vi "(C) Save to Excel (SubVI).vi"(0 "File Path Input":path, 1 "Save (Enable/Signal)":bool, 2 "Save Interval (s)":dbl=1.0, 3 "Title Block":string[][](array[string]), 4 "Column Header Array":string[](array[string]), 5 "Data Array (Row)":string[](array[string]), 7 "File Configuration":T1={"Row Limit"=65500, "Default File Name"="Data", "New File Daily?"=TRUE, "Manual Save Interval?"=FALSE}, 9 "Change Save Location?":bool, 11 "Reset Elapsed Time":bool caption="Reset Elapsed Time?") -> (14 "File Path Output":path, 15 "Save Indicator":bool, 16 "# of Rows Saved":i32, 17 "Elapsed Time":string="00:00:00", 19 "Error Output":errorcluster)   [LabVIEW 2010]
panel:
  # "SAVE TO EXCEL SUBVI\nSave 1D Array (Row) to File"
  # "Created by Blake Otting 3/7/2007\nLast Updated 4/15/2010"
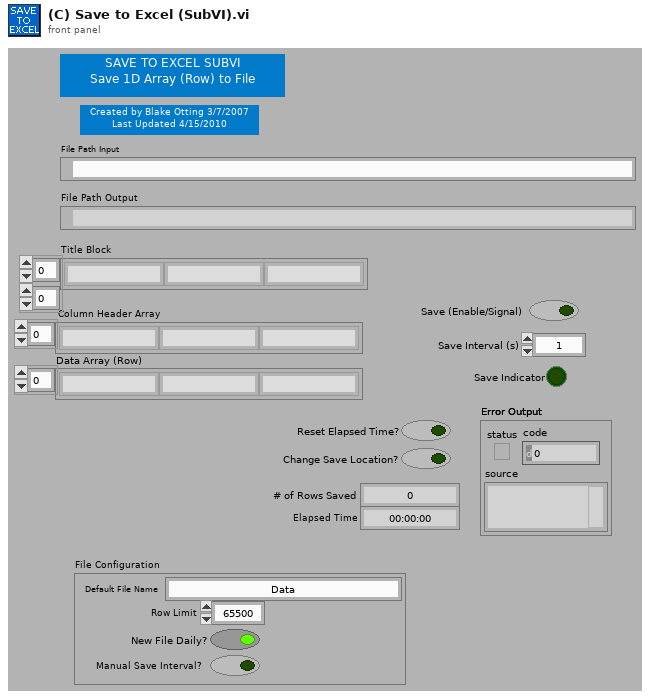
[diagram p1: front panel]
types:
  T1 = cluster{"Row Limit":i32, "Default File Name":string, "New File Daily?":bool, "Manual Save Interval?":bool}
  T2 = typedef "LVDateTimeRec.ctl" = cluster{"fractional second":dbl, "second":i32, "minute":i32, "hour":i32, "day of month":i32, "month":i32, "year":i32, "day of week":i32, "day of year":i32, "DST":i32}
  T3 = enum16{"open", "replace", "create", "open or create", "replace or create", "replace or create with confirmation"}
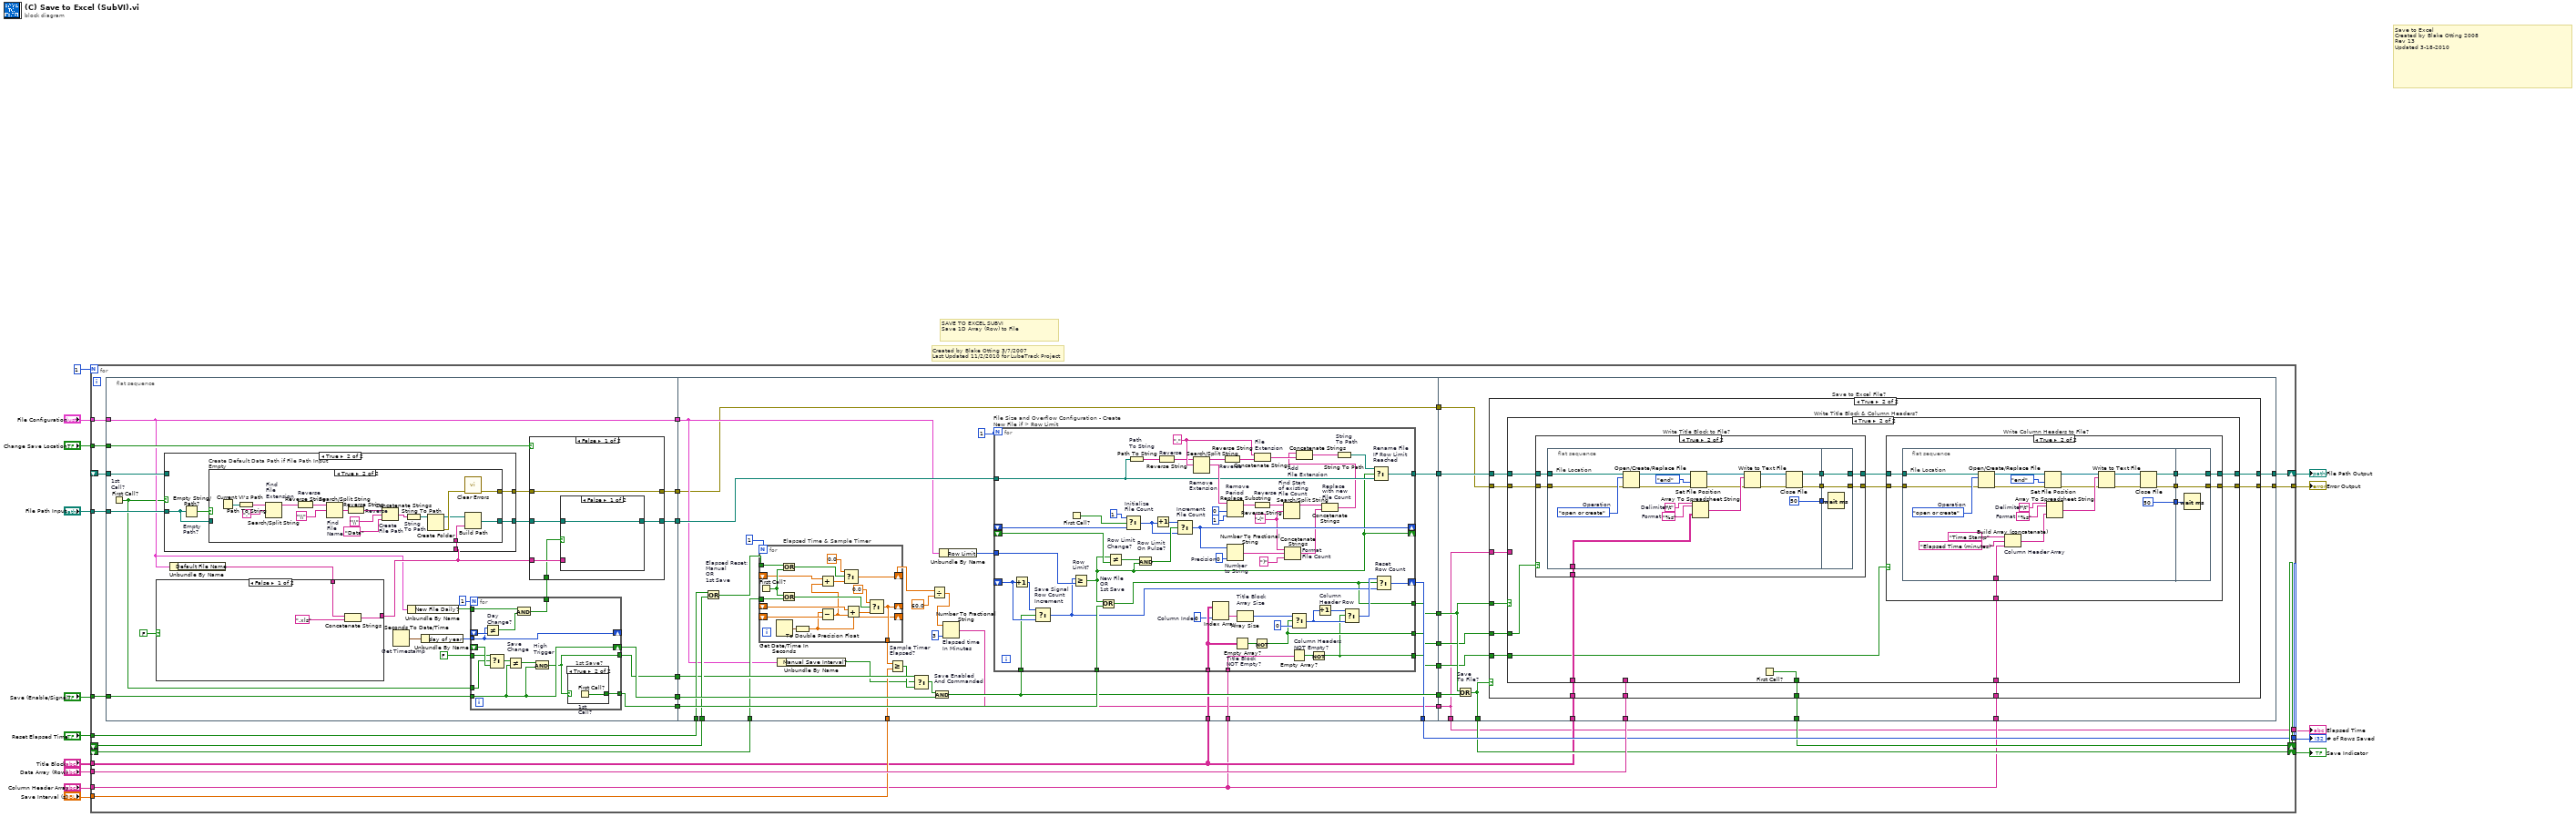
[diagram p0: block diagram]
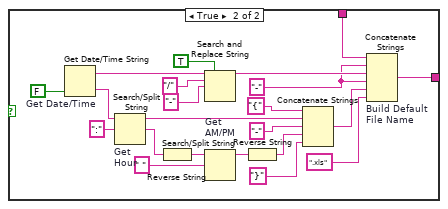
[diagram p2: hidden frame]
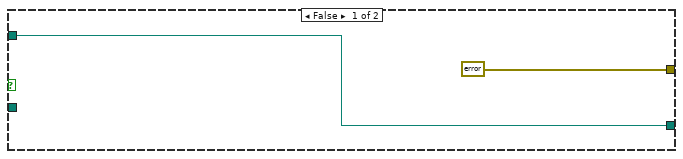
[diagram p4: hidden frame]
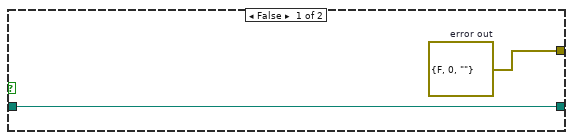
[diagram p5: hidden frame]
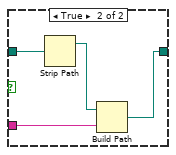
[diagram p6: hidden frame]
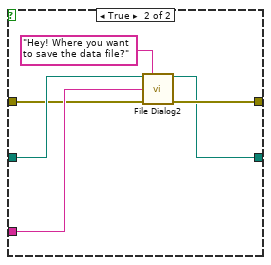
[diagram p7: hidden frame]
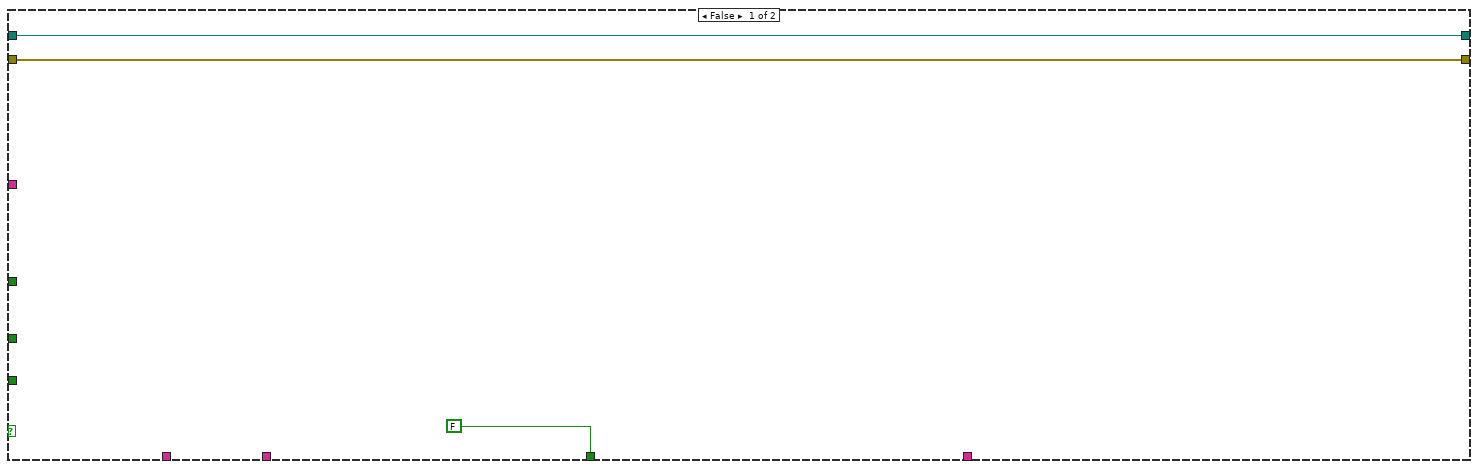
[diagram p8: hidden frame]
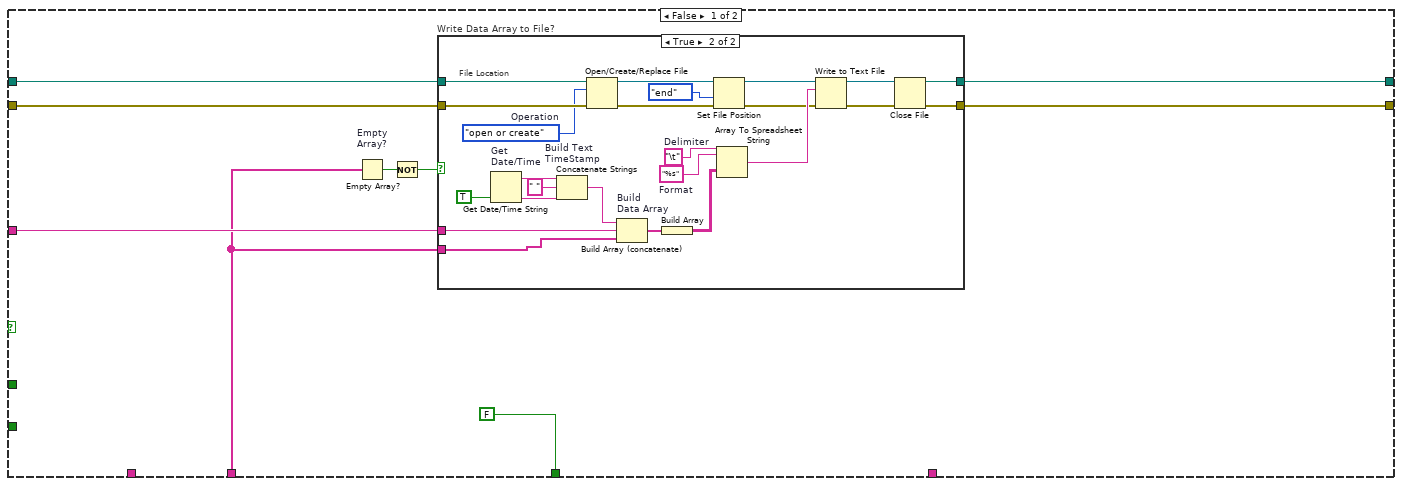
[diagram p9: hidden frame]
diagram:
  # "Created by Blake Otting 3/7/2007\nLast Updated 11/2/2010 for LubeTrack Project"
  # "SAVE TO EXCEL SUBVI\nSave 1D Array (Row) to File"
  # "Save to Excel\nCreated by Blake Otting 2008\nRev 13\nUpdated 3-18-2010"
  n1 = for {
    N: 1 -> [_]
    tunnel: "File Path Input" -> [w39]
    tunnel: "Change Save Location?" -> [w46]
    tunnel: "Save (Enable/Signal)" -> [w33]
    tunnel: "Data Array (Row)" -> [w40]
    tunnel: "Column Header Array" -> [w23]
    tunnel: "File Configuration" -> [w29]
    tunnel: "Reset Elapsed Time" -> [w30]
    shift-right: [w35] -> w14
    shift-left: _ -> [w43]
    tunnel: "Save Interval (s)" -> [w34]
    shift-right: [w36] -> _
    shift-left: _ -> [w31]
    tunnel: "Title Block" -> [w25]
    shift-right: [w41] -> w12
    shift-left: _ -> [w38]
    tunnel: [w19] -> w13
    tunnel: [w37] -> w15
    tunnel: [w26] -> w11
    n2 = flat-sequence {
      tunnel: w38 -> [w58]
      tunnel: w39 -> [w57]
      tunnel: w46 -> [w50]
      tunnel: w29 -> [w49]
      tunnel: [w52] -> w45
      tunnel: [w54] -> w44
      tunnel: w33 -> [w56]
      tunnel: [w55] -> w32
      tunnel: [w51] -> w28
      tunnel: [w49] -> w18
      tunnel: [w53] -> w17
      tunnel: [w180] -> w42
      tunnel: w43 -> [w163]
      tunnel: w44 -> [w154]
      tunnel: w45 -> [w181]
      tunnel: [w172] -> w37
      tunnel: w34 -> [w161]
      tunnel: w32 -> [w178]
      tunnel: w31 -> [w175]
      tunnel: w30 -> [w174]
      tunnel: w28 -> [w173]
      tunnel: [w154] -> w27
      tunnel: w25 -> [w171]
      tunnel: [w169] -> w24
      tunnel: w23 -> [w168]
      tunnel: [w167] -> w22
      tunnel: [w166] -> w21
      tunnel: [w159] -> w20
      tunnel: w18 -> [w158]
      tunnel: w17 -> [w170]
      tunnel: [w151] -> w16
      tunnel: w42 -> [w265]
      tunnel: [w263] -> w41
      tunnel: w25 -> [w262]
      tunnel: w40 -> [w261]
      tunnel: w23 -> [w260]
      tunnel: [w259] -> w35
      tunnel: [w258] -> w36
      tunnel: w27 -> [w257]
      tunnel: [w256] -> w26
      tunnel: w24 -> [w264]
      tunnel: w22 -> [w255]
      tunnel: w21 -> [w254]
      tunnel: w20 -> [w253]
      tunnel: [w252] -> w19
      tunnel: w16 -> [w252]
      frame #0 {
        n3 = First Call? "1st\nCall?"() -> (First Call?: T/F=w48:bool)
        n4 = Unbundle By Name(w49) -> ("Default File Name"=w60:string)
        n5 = case shown="False" FALSE {
          tunnel: [w69 w93] -> w68
          tunnel: w60 -> [w70 w92]
          frame False {
            n6 = Concatenate Strings(w70, ".xls" ("string")) -> (w69:string)
          }
          frame True {
            w81 = "-" ("string")
            n7 = Get Date/Time String "Get Date/Time"(want seconds? (F)=FALSE) -> (date string=w76:string, time string=w75:string)  [unwired: 2 out]
            n8 = Search/Split String "Get\nHour"(string=w75, search string/char (-)=":" ("search string")) -> (substring before match=w86:string, match + rest of string=w83:string)  [unwired: 2 out]
            n9 = Reverse String(1:w83) -> (0:w84:string)
            n10 = Search and Replace String(replace all?=TRUE ("replace all? (F)"), input string=w76, search string="/", replace string="-" ("replace string (\"\")")) -> (result string=w91:string)  [unwired: 1 in, 6 out]
            n11 = Search/Split String "Get\nAM/PM"(string=w84, search string/char (-)=" ") -> (substring before match=w85:string)  [unwired: 3 out]
            n12 = Reverse String(1:w85) -> (0:w87:string)
            n13 = Concatenate Strings ("Build\nHour String")("{" ("string"), w86, "-" ("search string/char (-)"), w87, "}" ("string")) -> (w78:string)
            n14 = Concatenate Strings "Build Default\nFile Name"(w92, w81, w91, w81, w78, ".xls" ("string")) -> (w93:string)
          }
        }
        n15 = case shown="True" w48 {
          tunnel: w57 -> [_ w114]
          tunnel: [w110 w113] -> w59
          tunnel: w68 -> [_ w112]
          tunnel: [errorcluster {"status"=FALSE, "code"=0, "source"=""} w111] -> w61
          tunnel: w58 -> [w110 _]
          frame False {
          }
          frame True {
            n16 = Empty String/Path? "Empty\nPath?"(string/path=w114) -> (empty?=w115:bool)
            n17 = case "Create Default Data Path if File Path Input Empty" shown="True" w115 {
              tunnel: [w117 w120] -> w113
              tunnel: w114 -> [w117 _]
              tunnel: w112 -> [_ w119]
              tunnel: [w116 w118] -> w111
              frame False {
                w116 = errorcluster {"status"=FALSE, "code"=0, "source"=""}  # error out
              }
              frame True {
                n18 = Current VI's Path() -> (path=w126:path)
                n19 = Path To String(path=w126) -> (string=w132:string)
                n20 = Search/Split String "Find\nFile \nExtension"(string=w132, search string/char (-)=".") -> (substring before match=w131:string)  [unwired: 1 in, 2 out]
                n21 = Reverse String "Reverse"(1:w131) -> (0:w130:string)
                n22 = Search/Split String "Find\nFile \nName"(string=w130, search string/char (-)="\\") -> (match + rest of string=w128:string)  [unwired: 1 in, 2 out]
                n23 = Reverse String "Reverse"(1:w128) -> (0:w127:string)
                n24 = Concatenate Strings "Create\nFile Path"(w127, "\\", "Data") -> (w134:string)
                n25 = String To Path "String\nTo Path"(string=w134) -> (path=w124:path)
                n26 = Create Folder(path (use dialog)=w124) -> (created path=w121:path, error out=w123:errorcluster)  [unwired: 2 in, 1 out]
                n27 = call <vilib>:"Clear Errors.vi"("error in (no error)"=w123) -> ("error out"=w118:errorcluster)  [unwired: 6 in]
                n28 = Build Path(base path=w121, name or relative path=w119) -> (appended path=w120:path)
              }
            }
          }
        }
        n29 = Seconds To Date/Time "Get Timestamp"() -> (date time rec=w66:T2)  [unwired: 2 out]
        n30 = Unbundle By Name(w49) -> ("New File Daily?"=w62:bool)
        n31 = Unbundle By Name(w66) -> ("day of year"=w63:i32)
        n32 = for {
          N: 1 -> [_]
          tunnel: w56 -> [w105]
          shift-right: [w105] -> w55
          shift-left: _ -> [w99]
          tunnel: w63 -> [w103]
          shift-right: [w103] -> _
          shift-left: _ -> [w104]
          tunnel: w62 -> [w101]
          tunnel: [w100] -> w65
          tunnel: [w97] -> w52
          tunnel: [w96] -> w51
          tunnel: w48 -> [w95]
          tunnel: FALSE -> [w94]
          n33 = Not Equal? "Day\nChange?"(x=w103, y=w104) -> (x != y?=w102:bool)
          n34 = Select(t=w94, s=w95, f=w99) -> (s? t:f=w98:bool)
          n35 = Not Equal? "Save\nChange"(x=w98, y=w105) -> (x != y?=w106:bool)
          n36 = And(x=w101, y=w102) -> (x .and. y?=w100:bool)
          n37 = And "High\nTrigger"(x=w106, y=w105) -> (x .and. y?=w96:bool)
          n38 = case "1st Save?" shown="True" w96 {
            selector: w96 -> [w107 _]
            tunnel: [w107 w108] -> w97
            frame False {
            }
            frame True {
              n39 = First Call? "1st\nCall?"() -> (First Call?: T/F=w108:bool)
            }
          }
        }
        n40 = case shown="False" w50 {
          tunnel: w59 -> [w138 w150]
          tunnel: w68 -> [w137 w148]
          tunnel: w61 -> [w139 w147]
          tunnel: [w139 w146] -> w54
          tunnel: w65 -> [w136 _]
          tunnel: [w135 w145] -> w53
          frame False {
            n41 = case shown="False" w136 {
              tunnel: w138 -> [w140 w144]
              tunnel: w137 -> [_ w142]
              tunnel: [w140 w141] -> w135
              frame False {
              }
              frame True {
                n42 = Strip Path(path=w144) -> (stripped path=w143:path)  [unwired: 1 out]
                n43 = Build Path(base path=w143, name or relative path=w142) -> (appended path=w141:path)
              }
            }
          }
          frame True {
            n44 = call "File Dialog2"("start path"=w150, "prompt"="Hey! Where you want to save the data file?", "default name"=w148, "error in"=w147) -> ("selected path"=w145:path, "error out"=w146:errorcluster)  [unwired: 3 in, 7 out]
          }
        }
      }
      frame #1 {
        n45 = Or "Elapsed Reset:\nManual\nOR\n1st Save"(x=w174, y=w175) -> (x .or. y?=w160:bool)
        n46 = for "Elapsed Time & Sample Timer" {
          N: 1 -> [_]
          shift-right: [w195] -> _
          shift-left: _ -> [w198]
          shift-right: [w187] -> _
          shift-left: _ -> [w197]
          tunnel: [w195] -> w164
          tunnel: w163 -> [w191]
          tunnel: w160 -> [w189]
          shift-right: [w183] -> w156
          shift-left: _ -> [w186]
          n47 = First Call?() -> (First Call?: T/F=w190:bool)
          n48 = Get Date/Time In Seconds() -> (seconds since 1Jan1904=w196:timestamp)
          n49 = Or(x=w189, y=w190) -> (x .or. y?=w184:bool)
          n50 = Or(x=w190, y=w191) -> (x .or. y?=w192:bool)
          n51 = To Double Precision Float(number=w196) -> (double precision float=w187:dbl)
          n52 = Subtract(x=w187, y=w197) -> (x-y=w182:dbl)
          n53 = Add(x=w186, y=w182) -> (x+y=w188:dbl)
          n54 = Select(t=0.0, s=w184, f=w188) -> (s? t:f=w183:dbl)
          n55 = Add(x=w198, y=w182) -> (x+y=w194:dbl)
          n56 = Select(t=0.0, s=w192, f=w194) -> (s? t:f=w195:dbl)
        }
        n57 = Unbundle By Name(w158) -> ("Manual Save Interval?"=w157:bool)
        n58 = Greater Or Equal? "Sample Timer\nElapsed?"(x=w164, y=w161) -> (x >= y?=w162:bool)
        n59 = Select(t=w173, s=w157, f=w162) -> (s? t:f=w179:bool)
        n60 = Divide(x=w156, y=60.0) -> (x/y=w152:dbl)
        n61 = And "Save Enabled\nAnd Commanded"(x=w179, y=w178) -> (x .and. y?=w180:bool)
        n62 = Unbundle By Name(w158) -> ("Row Limit"=w177:i32)
        n63 = Number To Fractional String "Elapsed time\nIn Minutes"(number=w152, precision (6)=i16 3) -> (F-format string=w151:string)  [unwired: 2 in]
        n64 = for "File Size and Overflow Configuration - Create New File if > Row Limit" {
          N: 1 -> [_]
          tunnel: w181 -> [w249]
          tunnel: w180 -> [w248]
          shift-right: [w246] -> w172
          shift-left: _ -> [w250]
          tunnel: w177 -> [w247]
          shift-right: [w214] -> _
          shift-left: _ -> [w245]
          tunnel: w171 -> [w201]
          shift-right: [w239] -> _
          shift-left: _ -> [w217]
          tunnel: w170 -> [w228]
          tunnel: [w220] -> w169
          tunnel: w168 -> [w212]
          tunnel: [w205] -> w166
          tunnel: [w204] -> w159
          tunnel: [w202] -> w167
          w200 = 0  # Column Index
          w237 = "." ("search string/char (-)")
          w221 = "-("
          w243 = i16 0  # Precision
          n65 = Increment(x=w250) -> (x+1=w251:i32)
          n66 = Select "Save Signal\nRow Count\nIncrement"(t=w251, s=w248, f=w250) -> (s? t:f=w203:i32)
          n67 = First Call?() -> (First Call?: T/F=w218:bool)
          n68 = Greater Or Equal? "Row\nLimit?"(x=w203, y=w247) -> (x >= y?=w214:bool)
          n69 = Or "New File\nOR\n1st Save"(x=w214, y=w249) -> (x .or. y?=w202:bool)
          n70 = Not Equal? "Row Limit\nChange?"(x=w214, y=w245) -> (x != y?=w240:bool)
          n71 = Select "Initialize\nFile Count"(t=i16 1, s=w218, f=w217) -> (s? t:f=w216:i16)
          n72 = Path To String "Path\nTo String"(path=w228) -> (string=w230:string)
          n73 = And "Row Limit\nOn Pulse?"(x=w240, y=w214) -> (x .and. y?=w244:bool)
          n74 = Increment(x=w216) -> (x+1=w241:i16)
          n75 = Reverse String "Reverse"(1:w230) -> (0:w231:string)
          n76 = Select "Increment\nFile Count"(t=w241, s=w244, f=w216) -> (s? t:f=w239:i16)
          n77 = Search/Split String "Remove\nExtension"(string=w231, search string/char (-)=w237) -> (substring before match=w232:string, match + rest of string=w233:string)  [unwired: 2 out]
          n78 = Index Array(array=w201, index (col)=w200) -> (element=w199:string[])  [unwired: 1 in]
          n79 = Reverse String "Reverse"(1:w232) -> (0:w229:string)
          n80 = Replace Substring "Remove\nPeriod"(2:1 ("length (len. of substring)"), 3:0 ("offset (0)"), 5:w233) -> (1:w234:string)  [unwired: 2 out]
          n81 = Number To Fractional String "Number\nto String"(number=w239, precision (6)=w243) -> (F-format string=w242:string)  [unwired: 2 in]
          n82 = Empty Array? "Title Block\nNOT Empty?"(array=w201) -> (empty?=w211:bool)
          n83 = Array Size "Title Block\nArray Size"(array=w199) -> (size(s)=w210:i32)
          n84 = Reverse String "Reverse"(1:w234) -> (0:w226:string)
          n85 = Not(x=w211) -> (.not. x?=w205:bool)
          n86 = Concatenate Strings "File\nExtension"(w237, w229) -> (w223:string)
          n87 = Search/Split String "Find Start\nof existing\nFile Count"(string=w226, search string/char (-)=w221) -> (substring before match=w225:string)  [unwired: 1 in, 2 out]
          n88 = Concatenate Strings "Format\nFile Count"(w221, w242, ")") -> (w224:string)
          n89 = Empty Array? "Column Headers\nNOT Empty?"(array=w212) -> (empty?=w213:bool)
          n90 = Select(t=w210, s=w205, f=0 ("t")) -> (s? t:f=w208:i32)
          n91 = Not(x=w213) -> (.not. x?=w204:bool)
          n92 = Increment "Column\nHeader Row"(x=w208) -> (x+1=w207:i32)
          n93 = Concatenate Strings "Replace\nwith new\nFile Count"(w225, w224) -> (w215:string)
          n94 = Concatenate Strings "Add\nFile Extension"(w215, w223) -> (w222:string)
          n95 = String To Path "String\nTo Path"(string=w222) -> (path=w238:path)
          n96 = Select(t=w207, s=w204, f=w208) -> (s? t:f=w206:i32)
          n97 = Select "Rename File\nIF Row Limit\nReached"(t=w238, s=w214, f=w228) -> (s? t:f=w220:path)
          n98 = Select "Reset\nRow Count"(t=w206, s=w202, f=w203) -> (s? t:f=w246:i32)
        }
      }
      frame #2 {
        n99 = Or "Save\nTo File?"(x=w255, y=w265) -> (x .or. y?=w259:bool)
        n100 = case "Save to Excel File?" shown="True" w259 {
          tunnel: [w268 w280] -> w263
          tunnel: w264 -> [w268 w279]
          tunnel: w255 -> [_ w278]
          tunnel: [FALSE ("First Call?: T/F") w277] -> w258
          tunnel: w252 -> [_ w276]
          tunnel: w262 -> [_ w273]
          tunnel: w261 -> [_ w275]
          tunnel: w260 -> [_ w274]
          tunnel: w257 -> [w266 w272]
          tunnel: [w266 w271] -> w256
          tunnel: w254 -> [_ w270]
          tunnel: w253 -> [_ w269]
          frame False {
          }
          frame True {
            n101 = case "Write Title Block & Column Headers?" shown="True" w278 {
              tunnel: [w287 w321] -> w280
              tunnel: w279 -> [w288 w325]
              tunnel: w273 -> [_ w319]
              tunnel: w274 -> [_ w318]
              tunnel: w276 -> [w286 _]
              tunnel: [FALSE ("First Call?: T/F") w326] -> w277
              tunnel: w275 -> [w282 _]
              tunnel: w272 -> [w285 w322]
              tunnel: [w284 w320] -> w271
              tunnel: w270 -> [_ w317]
              tunnel: w269 -> [_ w316]
              frame False {
                n102 = Empty Array? "Empty\nArray?"(array=w282) -> (empty?=w283:bool)
                n103 = Not(x=w283) -> (.not. x?=w281:bool)
                n104 = case "Write Data Array to File?" shown="True" w281 {
                  tunnel: w288 -> [w291 w315]
                  tunnel: [w291 w314] -> w287
                  tunnel: w282 -> [_ w292]
                  tunnel: w286 -> [_ w293]
                  tunnel: w285 -> [w290 w313]
                  tunnel: [w290 w312] -> w284
                  frame False {
                  }
                  frame True {
                    w301 = "\t"  # Delimiter
                    w300 = "%s"  # Format
                    w308 = T3."open or create"  # Operation
                    # "File Location"
                    n105 = Get Date/Time String "Get \nDate/Time"(want seconds? (F)=TRUE) -> (date string=w303:string, time string=w306:string)  [unwired: 2 out]
                    n106 = Concatenate Strings "Build Text\nTimeStamp"(w303, " " ("string"), w306) -> (w307:string)
                    n107 = Open/Create/Replace File(file path (use dialog)=w315, error in=w313, operation (0:open)=w308) -> (refnum out=w294:refnum<file>, error out=w295:errorcluster)  [unwired: 3 in, 1 out]
                    n108 = Build Array (concatenate) "Build\nData Array"(w307, w293, w292) -> (w310:string[])
                    n109 = Build Array(w310) -> (w311:string[][])
                    n110 = Set File Position(refnum=w294, from (0:start)=enum16{"start", "end", "current"}."end", error in=w295) -> (refnum out=w296:refnum<file>, error out=w297:errorcluster)  [unwired: 1 in]
                    n111 = Array To Spreadsheet String(delimiter (Tab)=w301, array=w311, 3:w300) -> (spreadsheet string=w302:string)
                    n112 = Write to Text File(file (use dialog)=w296, text=w302, error in=w297) -> (refnum out=w298:refnum<file>, error out=w299:errorcluster)  [unwired: 1 in, 1 out]
                    n113 = Close File(refnum=w298, error in=w299) -> (path=w314:path, error out=w312:errorcluster)
                  }
                }
              }
              frame True {
                n114 = case "Write Title Block to File?" shown="True" w317 {
                  tunnel: w325 -> [w360 w369]
                  tunnel: w319 -> [_ w368]
                  tunnel: [w361 w367] -> w323
                  tunnel: [w360 w366] -> w324
                  tunnel: w322 -> [w361 w365]
                  frame False {
                  }
                  frame True {
                    n115 = flat-sequence "Write to Excel File" {
                      tunnel: w368 -> [w370]
                      tunnel: w369 -> [w375]
                      tunnel: w365 -> [w372]
                      tunnel: [w374] -> w364
                      tunnel: [w373] -> w363
                      tunnel: [u32 50 ("milliseconds to wait")] -> w362
                      tunnel: [w388] -> w367
                      tunnel: [w389] -> w366
                      tunnel: w364 -> [w389]
                      tunnel: w363 -> [w388]
                      tunnel: w362 -> [w387]
                      frame #0 {
                        w383 = "\t"  # Delimiter
                        w382 = "%s"  # Format
                        w385 = T3."open or create"  # Operation
                        # "File Location"
                        n116 = Open/Create/Replace File(file path (use dialog)=w375, error in=w372, operation (0:open)=w385) -> (refnum out=w376:refnum<file>, error out=w377:errorcluster)  [unwired: 3 in, 1 out]
                        n117 = Set File Position(refnum=w376, from (0:start)=enum16{"start", "end", "current"}."end", error in=w377) -> (refnum out=w378:refnum<file>, error out=w379:errorcluster)  [unwired: 1 in]
                        n118 = Array To Spreadsheet String(delimiter (Tab)=w383, array=w370, 3:w382) -> (spreadsheet string=w384:string)
                        n119 = Write to Text File(file (use dialog)=w378, text=w384, error in=w379) -> (refnum out=w380:refnum<file>, error out=w381:errorcluster)  [unwired: 1 in, 1 out]
                        n120 = Close File(refnum=w380, error in=w381) -> (path=w374:path, error out=w373:errorcluster)
                      }
                      frame #1 {
                        n121 = Wait (ms)(milliseconds to wait=w387) -> ()  [unwired: 1 out]
                      }
                    }
                  }
                }
                n122 = First Call?() -> (First Call?: T/F=w326:bool)
                n123 = case "Write Column Headers to File?" shown="True" w316 {
                  tunnel: w324 -> [w327 w336]
                  tunnel: [w328 w335] -> w320
                  tunnel: w323 -> [w328 w334]
                  tunnel: [w327 w333] -> w321
                  tunnel: w318 -> [_ w332]
                  frame False {
                  }
                  frame True {
                    n124 = flat-sequence "Write to Excel File" {
                      tunnel: w336 -> [w345]
                      tunnel: w334 -> [w342]
                      tunnel: w332 -> [w337]
                      tunnel: [w344] -> w331
                      tunnel: [w343] -> w330
                      tunnel: [u32 50 ("milliseconds to wait")] -> w329
                      tunnel: [w358] -> w335
                      tunnel: [w359] -> w333
                      tunnel: w331 -> [w359]
                      tunnel: w330 -> [w358]
                      tunnel: w329 -> [w357]
                      frame #0 {
                        w353 = "\t"  # Delimiter
                        w352 = "%s"  # Format
                        w355 = T3."open or create"  # Operation
                        # "File Location"
                        n125 = Open/Create/Replace File(file path (use dialog)=w345, error in=w342, operation (0:open)=w355) -> (refnum out=w346:refnum<file>, error out=w347:errorcluster)  [unwired: 3 in, 1 out]
                        n126 = Build Array (concatenate) "Column Header Array"("Time Stamp", "Elapsed Time (minutes)", w337) -> (w340:string[])
                        n127 = Set File Position(refnum=w346, from (0:start)=enum16{"start", "end", "current"}."end", error in=w347) -> (refnum out=w348:refnum<file>, error out=w349:errorcluster)  [unwired: 1 in]
                        n128 = Array To Spreadsheet String(delimiter (Tab)=w353, array=w340, 3:w352) -> (spreadsheet string=w354:string)
                        n129 = Write to Text File(file (use dialog)=w348, text=w354, error in=w349) -> (refnum out=w350:refnum<file>, error out=w351:errorcluster)  [unwired: 1 in, 1 out]
                        n130 = Close File(refnum=w350, error in=w351) -> (path=w344:path, error out=w343:errorcluster)
                      }
                      frame #1 {
                        n131 = Wait (ms)(milliseconds to wait=w357) -> ()  [unwired: 1 out]
                      }
                    }
                  }
                }
              }
            }
          }
        }
      }
    }
  }
  "# of Rows Saved" <- w15
  "Save Indicator" <- w14
  "File Path Output" <- w12
  "Error Output" <- w11
  "Elapsed Time" <- w13
